vi "data parsing(debug2) from csv.vi"(11 "배열":string[](array[string])) -> (0 "Temp":u32[](array[numeric]), 1 "Filtered Sensor":u32[][](array[numeric]), 2 "No Filter Sensor":u32[][](array[numeric]), 3 "Time":string[](array[string]))   [LabVIEW 2015]
panel:
  out "Filtered Sensor 6":u32[](array[numeric])
  out "Filtered Sensor 5":u32[](array[numeric])
  out "Filtered Sensor 4":u32[](array[numeric])
  out "Filtered Sensor 3":u32[](array[numeric])
  out "Filtered Sensor 2":u32[](array[numeric])
  out "Filtered Sensor 1":u32[](array[numeric])
  out "No Filter Sensor 6":u32[](array[numeric])
  out "No Filter Sensor 5":u32[](array[numeric])
  out "No Filter Sensor 4":u32[](array[numeric])
  out "No Filter Sensor 3":u32[](array[numeric])
  out "No Filter Sensor 2":u32[](array[numeric])
  out "No Filter Sensor 1":u32[](array[numeric])
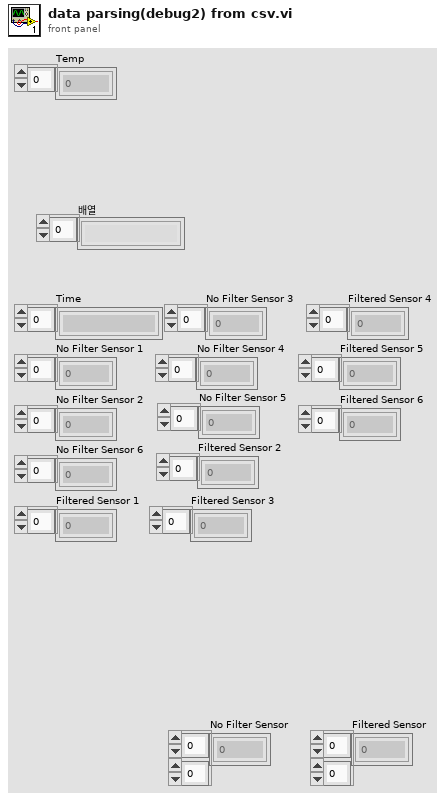
[diagram p1: front panel]
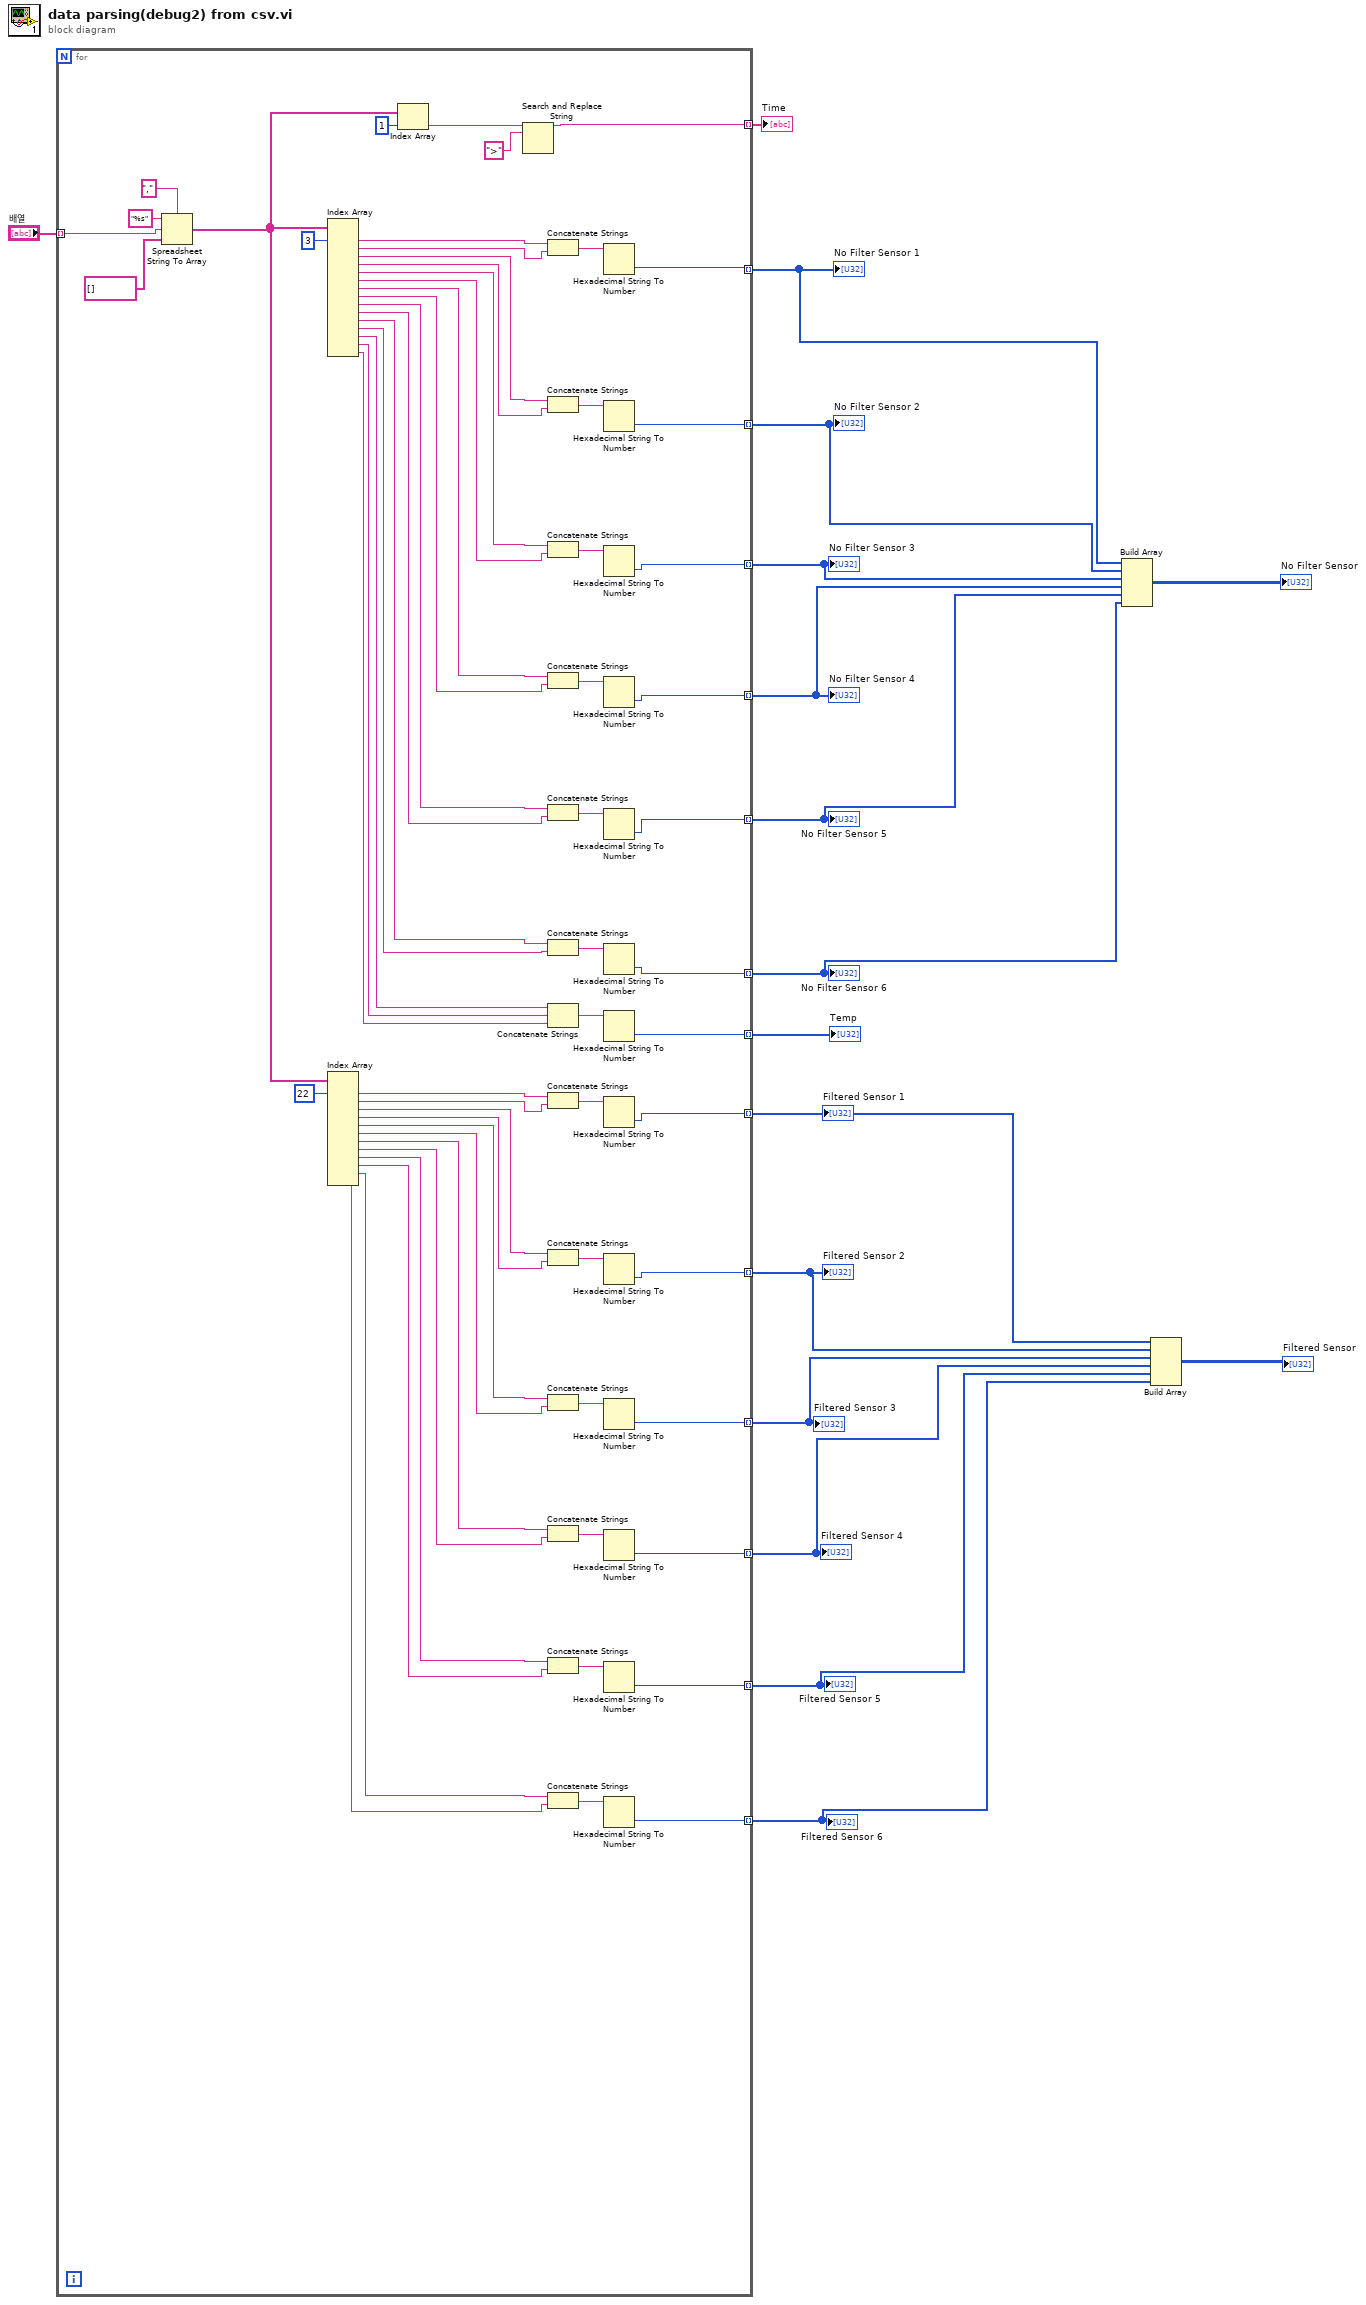
[diagram p0: block diagram]
diagram:
  n1 = for {
    tunnel: "배열" -> [w68] mode=indexing
    tunnel: [w47] -> w16 mode=indexing
    tunnel: [w34] -> w13 mode=indexing
    tunnel: [w33] -> w14 mode=indexing
    tunnel: [w32] -> w15 mode=indexing
    tunnel: [w31] -> w12 mode=indexing
    tunnel: [w30] -> w11 mode=indexing
    tunnel: [w29] -> w10 mode=indexing
    tunnel: [w28] -> w7 mode=indexing
    tunnel: [w27] -> w6 mode=indexing
    tunnel: [w26] -> w5 mode=indexing
    tunnel: [w25] -> w4 mode=indexing
    tunnel: [w24] -> w3 mode=indexing
    tunnel: [w23] -> w2 mode=indexing
    tunnel: [w18] -> w1 mode=indexing
    n2 = Spreadsheet String To Array(delimiter (Tab)="," ("구분 문자(탭)"), format string="%s" ("포맷 문자열"), spreadsheet string=w68, array type (2D Dbl)=string[] []) -> (array=w49:string[])
    n3 = Index Array(array=w49, index #1=3 ("비활성화된 인덱스 (열)")) -> (element #1=w81:string, element #2=w80:string, element #3=w79:string, element #4=w78:string, element #5=w77:string, element #6=w76:string, element #7=w75:string, element #8=w74:string, element #9=w73:string, element #10=w72:string, element #11=w64:string, element #12=w63:string, element #13=w21:string, element #14=w20:string, element #15=w19:string)  [unwired: 14 in]
    n4 = Index Array(array=w49, index #1=22 ("비활성화된 인덱스 (열)")) -> (element #1=w50:string, element #2=w51:string, element #3=w52:string, element #4=w53:string, element #5=w54:string, element #6=w55:string, element #7=w56:string, element #8=w57:string, element #9=w58:string, element #10=w59:string, element #11=w61:string, element #12=w62:string)  [unwired: 11 in]
    n5 = Index Array(array=w49, index=1 ("비활성화된 인덱스 (열)")) -> (element=w71:string)
    n6 = Search and Replace String(input string=w71, search string=">" ("검색 문자열")) -> (result string=w47:string)  [unwired: 6 in, 3 out]
    n7 = Concatenate Strings(w81, w80) -> (w46:string)
    n8 = Concatenate Strings(w79, w78) -> (w45:string)
    n9 = Concatenate Strings(w77, w76) -> (w44:string)
    n10 = Concatenate Strings(w75, w74) -> (w43:string)
    n11 = Concatenate Strings(w73, w72) -> (w42:string)
    n12 = Concatenate Strings(w64, w63) -> (w41:string)
    n13 = Concatenate Strings(w21, w20, w19) -> (w22:string)
    n14 = Concatenate Strings(w50, w51) -> (w40:string)
    n15 = Concatenate Strings(w52, w53) -> (w38:string)
    n16 = Concatenate Strings(w54, w55) -> (w39:string)
    n17 = Concatenate Strings(w56, w57) -> (w37:string)
    n18 = Concatenate Strings(w58, w59) -> (w36:string)
    n19 = Concatenate Strings(w61, w62) -> (w35:string)
    n20 = Hexadecimal String To Number(string=w46) -> (number=w34:u32)  [unwired: 2 in, 1 out]
    n21 = Hexadecimal String To Number(string=w45) -> (number=w33:u32)  [unwired: 2 in, 1 out]
    n22 = Hexadecimal String To Number(string=w44) -> (number=w32:u32)  [unwired: 2 in, 1 out]
    n23 = Hexadecimal String To Number(string=w43) -> (number=w31:u32)  [unwired: 2 in, 1 out]
    n24 = Hexadecimal String To Number(string=w42) -> (number=w30:u32)  [unwired: 2 in, 1 out]
    n25 = Hexadecimal String To Number(string=w41) -> (number=w29:u32)  [unwired: 2 in, 1 out]
    n26 = Hexadecimal String To Number(string=w22) -> (number=w18:u32)  [unwired: 2 in, 1 out]
    n27 = Hexadecimal String To Number(string=w40) -> (number=w28:u32)  [unwired: 2 in, 1 out]
    n28 = Hexadecimal String To Number(string=w38) -> (number=w27:u32)  [unwired: 2 in, 1 out]
    n29 = Hexadecimal String To Number(string=w39) -> (number=w26:u32)  [unwired: 2 in, 1 out]
    n30 = Hexadecimal String To Number(string=w37) -> (number=w25:u32)  [unwired: 2 in, 1 out]
    n31 = Hexadecimal String To Number(string=w36) -> (number=w24:u32)  [unwired: 2 in, 1 out]
    n32 = Hexadecimal String To Number(string=w35) -> (number=w23:u32)  [unwired: 2 in, 1 out]
  }
  "Time" <- w16
  "No Filter Sensor 1" <- w13
  "No Filter Sensor 2" <- w14
  "No Filter Sensor 3" <- w15
  "No Filter Sensor 4" <- w12
  "No Filter Sensor 5" <- w11
  "No Filter Sensor 6" <- w10
  "Filtered Sensor 1" <- w7
  "Filtered Sensor 2" <- w6
  "Filtered Sensor 3" <- w5
  "Filtered Sensor 4" <- w4
  "Filtered Sensor 5" <- w3
  "Filtered Sensor 6" <- w2
  "Temp" <- w1
  n33 = Build Array(w13, w14, w15, w12, w11, w10) -> (→"No Filter Sensor":u32[][])
  n34 = Build Array(w7, w6, w5, w4, w3, w2) -> (→"Filtered Sensor":u32[][])
